vi "hw2.6.vi"() -> ()   [LabVIEW 2014]
panel:
  out "combination":i32[](array[numeric])
  out "total combination":dbl
  out "probability":i32[](array[numeric])
  out "6.3":cluster{i32[], dbl[]}(graph)
  out "6.2":cluster{i32[], i32[]}(graph)
  out "Array 3":cluster{i32, i32[][]}[](array[cluster])
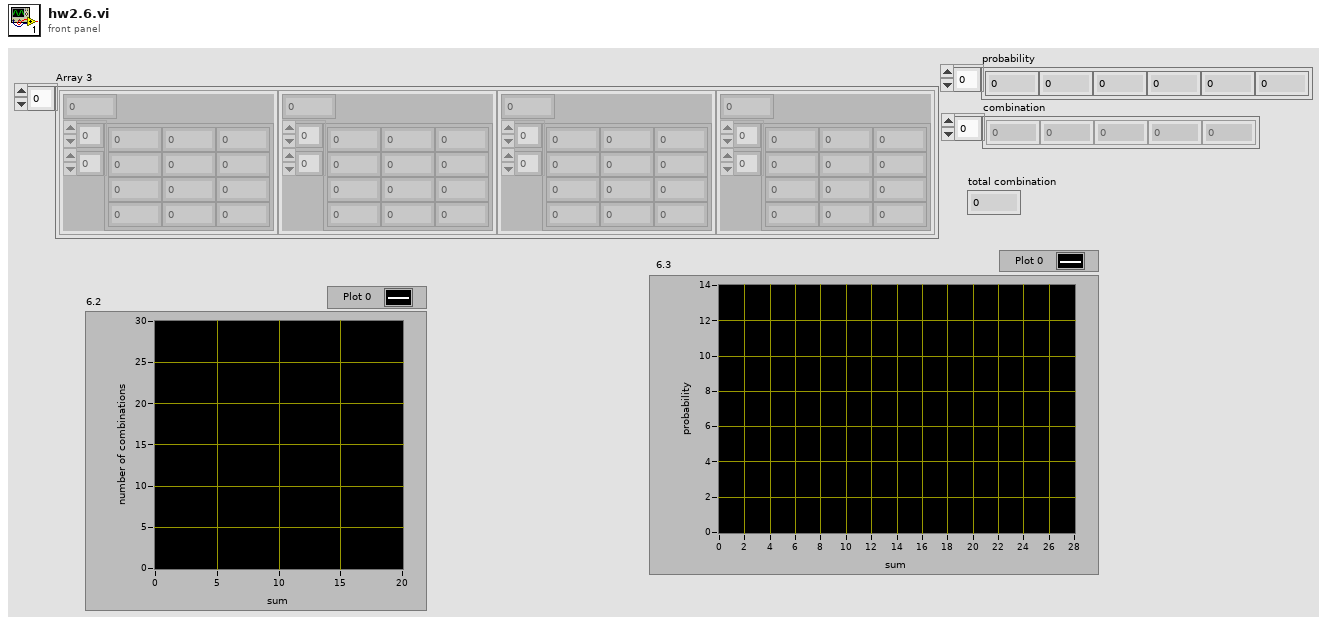
[diagram p1: front panel]
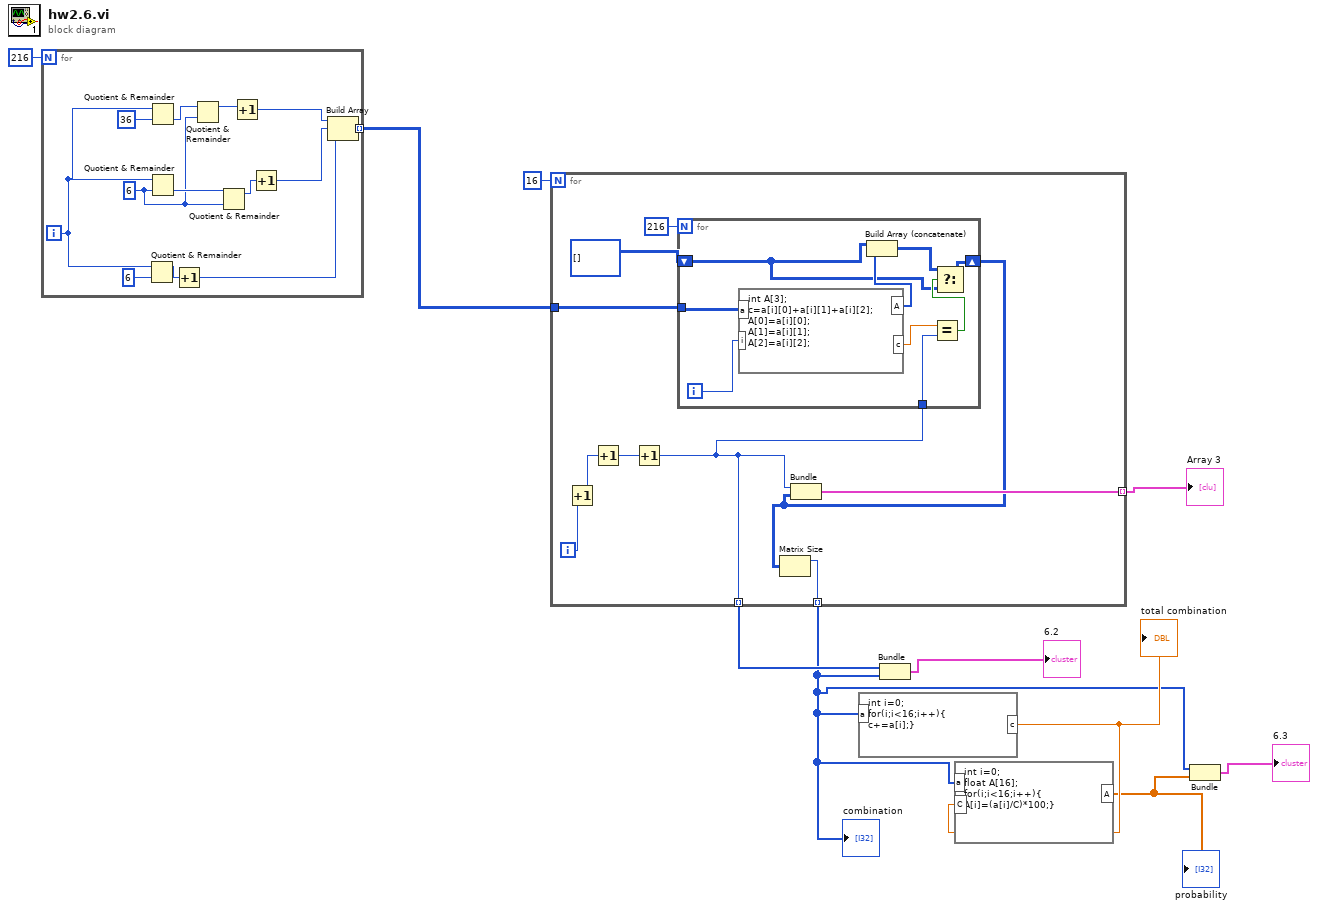
[diagram p0: block diagram]
diagram:
  n1 = for {
    N: 216 -> [_]
    tunnel: [w20] -> w8 mode=indexing
    i -> [w22]
    w12 = 6 ("y")
    n2 = Quotient & Remainder(x=w22, y=6) -> (x-y*floor(x/y)=w16:i32)  [unwired: 1 out]
    n3 = Quotient & Remainder(x=w22, y=36) -> (floor(x/y)=w13:i32)  [unwired: 1 out]
    n4 = Quotient & Remainder(x=w22, y=w12) -> (floor(x/y)=w15:i32)  [unwired: 1 out]
    n5 = Increment(x=w16) -> (x+1=w19:i32)
    n6 = Quotient & Remainder(x=w13, y=w12) -> (x-y*floor(x/y)=w11:i32)  [unwired: 1 out]
    n7 = Quotient & Remainder(x=w15, y=w12) -> (x-y*floor(x/y)=w14:i32)  [unwired: 1 out]
    n8 = Increment(x=w11) -> (x+1=w17:i32)
    n9 = Increment(x=w14) -> (x+1=w18:i32)
    n10 = Build Array(w17, w18, w19) -> (w20:i32[])
  }
  n11 = for {
    N: 16 -> [_]
    tunnel: w8 -> [w31]
    tunnel: [w29] -> w7 mode=indexing
    tunnel: [w25] -> w2 mode=indexing
    tunnel: [w24] -> w6 mode=indexing
    i -> [w33]
    n12 = Increment(x=w33) -> (x+1=w27:i32)
    n13 = Increment(x=w27) -> (x+1=w28:i32)
    n14 = Increment(x=w28) -> (x+1=w24:i32)
    n15 = for {
      N: 216 -> [_]
      tunnel: w31 -> [w42]
      shift-right: [w35] -> w26
      shift-left: i32[][] [] -> [w34]
      tunnel: w24 -> [w37]
      i -> [w41]
      n16 = formula code="int A[3];\nc=a[i][0]+a[i][1]+a[i][2];\nA[0]=a[i][0];\nA[1]=a[i][1];\nA[2]=a[i][2];"("a"=w42, "i"=w41) -> ("c"=w38:dbl, "A"=w40:i32[])
      n17 = Build Array (concatenate)(w34, w40) -> (w39:i32[][])
      n18 = Equal?(x=w38, y=w37) -> (x = y?=w36:bool)
      n19 = Select(t=w39, s=w36, f=w34) -> (s? t:f=w35:i32[][])
    }
    n20 = Matrix Size(0:w26) -> (1:w25:i32)  [unwired: 1 out]
    n21 = Bundle(w24, w26) -> (w29:cluster{i32, i32[][]})  [unwired: 1 in]
  }
  "Array 3" <- w7
  "combination" <- w2
  n22 = formula code="int i=0;\nfor(i;i<16;i++){\nc+=a[i];}"("a"=w2) -> ("c"=w4:dbl)
  "total combination" <- w4
  n23 = Bundle(w6, w2) -> (→"6.2":cluster{i32[], i32[]})  [unwired: 1 in]
  n24 = formula code="int i=0;\nfloat A[16];\nfor(i;i<16;i++){\nA[i]=(a[i]/C)*100;}"("a"=w2, "C"=w4) -> ("A"=w3:dbl[])
  "probability" <- w3
  n25 = Bundle(w2, w3) -> (→"6.3":cluster{i32[], dbl[]})  [unwired: 1 in]
